vi "Write Timeout.vi"(8 "error in (no error)":errorcluster, 10 "Timeout":i32, 11 "Wait On Boolean Step Config in":refnum<class "Wait On Boolean Step Config.lvclass">) -> (0 "error out":errorcluster, 3 "Wait On Boolean Step Config out":refnum<class "Wait On Boolean Step Config.lvclass">)   [LabVIEW 2015, in "Wait On Boolean Step Config.lvclass"]
uses:
  Wait On Boolean Step Config.lvclass
  Wait On Boolean Step Config.lvclass/Wait On Boolean Step Config.ctl
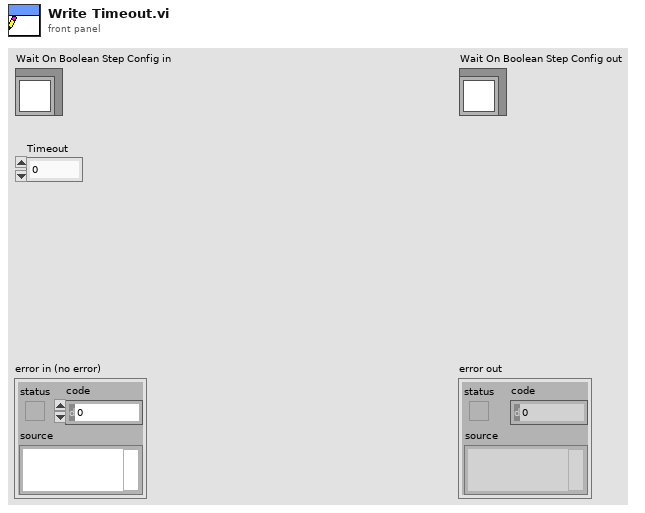
[diagram p1: front panel]
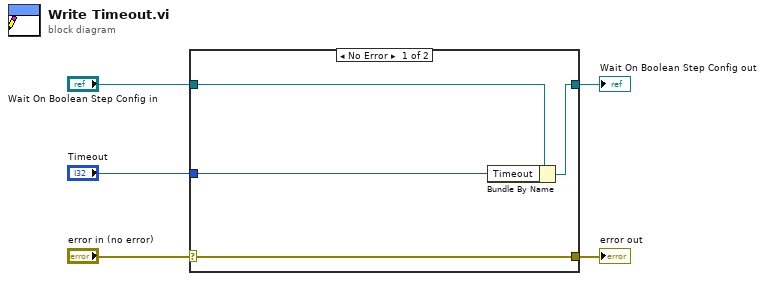
[diagram p0: block diagram]
diagram:
  n1 = case shown="No Error" "error in (no error)" {
    selector: "error in (no error)" -> [w9 w10]
    tunnel: [w9 w10] -> w4
    tunnel: [w7 w11] -> w2
    tunnel: "Wait On Boolean Step Config in" -> [w8 w11]
    tunnel: "Timeout" -> [w6 _]
    frame No Error {
      n2 = Bundle By Name(cluster=w8, "Timeout"=w6) -> (w7:refnum<class "Wait On Boolean Step Config.lvclass">)
    }
    frame Error {
    }
  }
  "error out" <- w4
  "Wait On Boolean Step Config out" <- w2
